vi "mirrorInterface.vi"(8 "error in (no error)":errorcluster, 11 "FPGA VI In":refnum<k20>) -> (0 "error out":errorcluster, 3 "FPGA VI Reference Out":refnum<k20>)   [LabVIEW 2016]
uses:
  controls/SocketServerStates.ctl
  <vilib>/Platform/TimedLoop/XDataNode/timing_clust.ctl
  <vilib>/Platform/TimedLoop/XDataNode/nitl_modes.ctl
  <vilib>/Platform/TimedLoop/XDataNode/wakeup.ctl
  <vilib>/Utility/error.llb/Error Cluster From Error Code.vi
  <vilib>/rvi/errors/niLvFpgaAdjustHostInterfaceError.vi
  <vilib>/platform/TimedLoop/XDataNode/XDataNode.xnode
  <vilib>/rvi/interface/nirviMethod/nirviMethod.xnode
  <vilib>/rvi/errors/niLvFpgaMergeErrorWithErrorCode.vi
  <vilib>/Platform/TimedLoop/XDataNode/XDNodeRunTimeDep.lvlib
  <vilib>/FPGAPlugInAG/Dynamic/niLvFpga_WriteFifo_Dynamic.vi
  controls/RT-Variables.lvlib
panel:
  out "bytes written 2":i32
  out "bytes written":i32
  out "length":i32
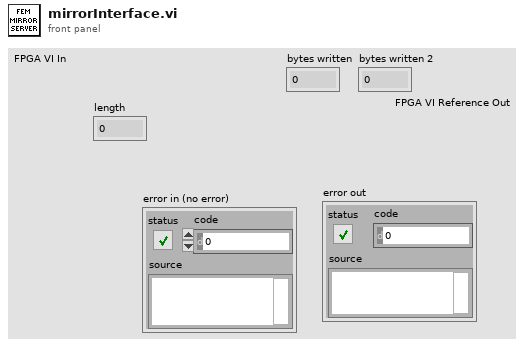
[diagram p1: front panel]
types:
  T1 = typedef "RT-Variables.lvlib/SocketServerStates.ctl" = enum16{"Wait", "SwitchState", "SingleUpdate", "ClosedLoop", "GetValues", "Exit"}
  T2 = typedef "XDNodeRunTimeDep.lvlib/timing_clust.ctl" = cluster{"Expected End [f-1]":u64, "Actual End [f-1]":u64, "Finished Late? [f-1]":bool, "Expected End [i-1]":u64, "Actual End [i-1]":u64, "Finished Late? [i-1]":bool, "Expected Start [i]":u64, "Actual Start [i]":u64, "Expected Start [f]":u64, "Actual Start [f]":u64, "Source Name":string, "Structure Name":string, "Period":i64, "Deadline":i64, "Offset":i64, "Start":i64, "Priority":i32, "Timeout":i32, "Mode":T3, "Wakeup Reason":T4, "Error":errorcluster, "Source Type":string, "Secondary Source Type":string, "Global End Time":u64, "Global Start Time":u64, "Frame Duration":u64, "Iteration Duration":u64, "Assigned CPU":i32, "I/O Scan Engine Mode":u32}
  T3 = typedef "XDNodeRunTimeDep.lvlib/nitl_modes.ctl" = enum32{"No Change", "Process missed periods, maintain original phase", "Discard missed periods, maintain original phase", "Process missed periods, ignore original phase", "Discard missed periods, ignore original phase"}
  T4 = typedef "XDNodeRunTimeDep.lvlib/wakeup.ctl" = enum32{"Normal", "Aborted", "Asynchronous wakeup", "Timing source error", "Timed loop error", "Timeout"}
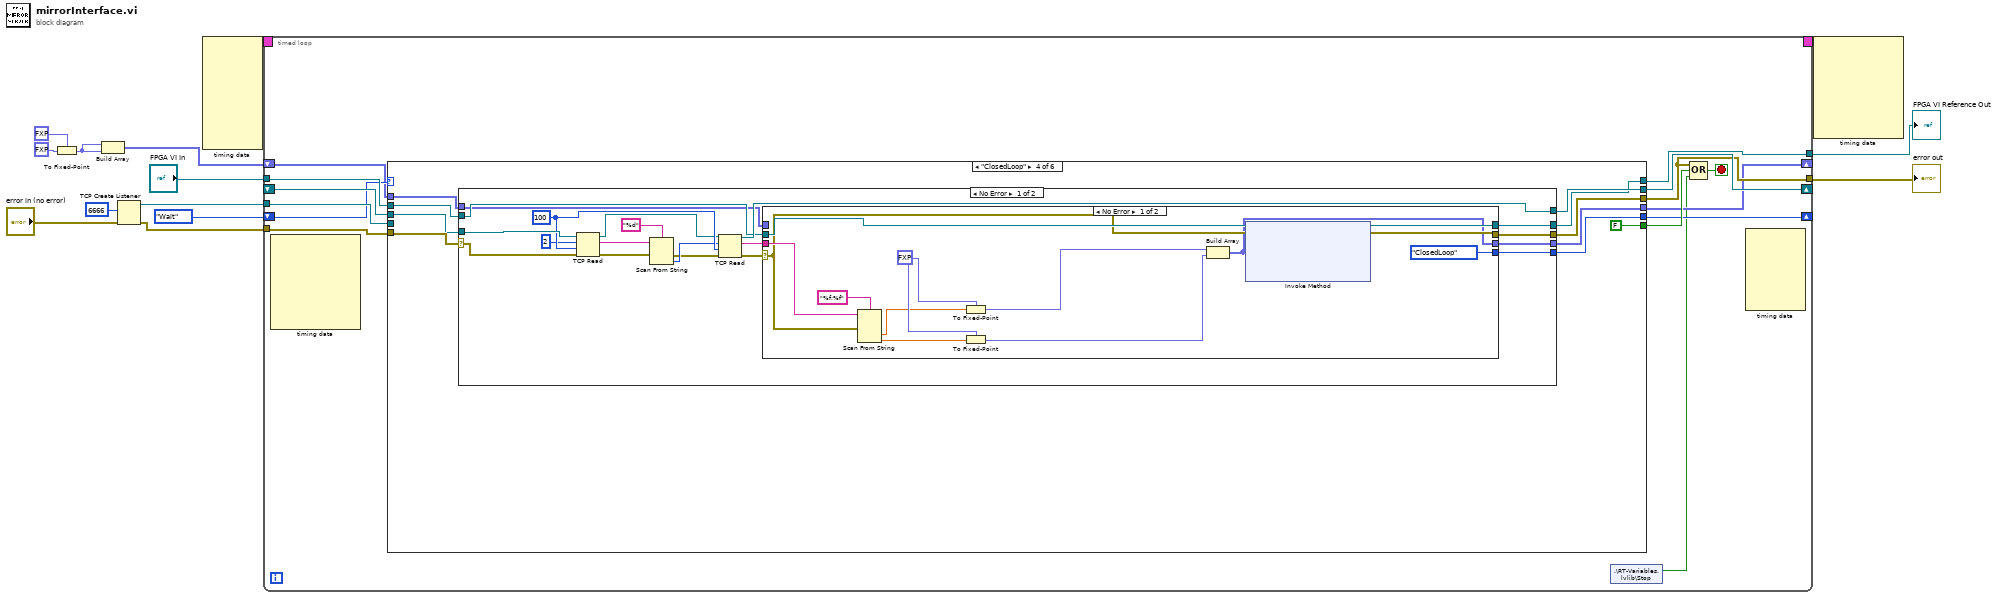
[diagram p0: block diagram]
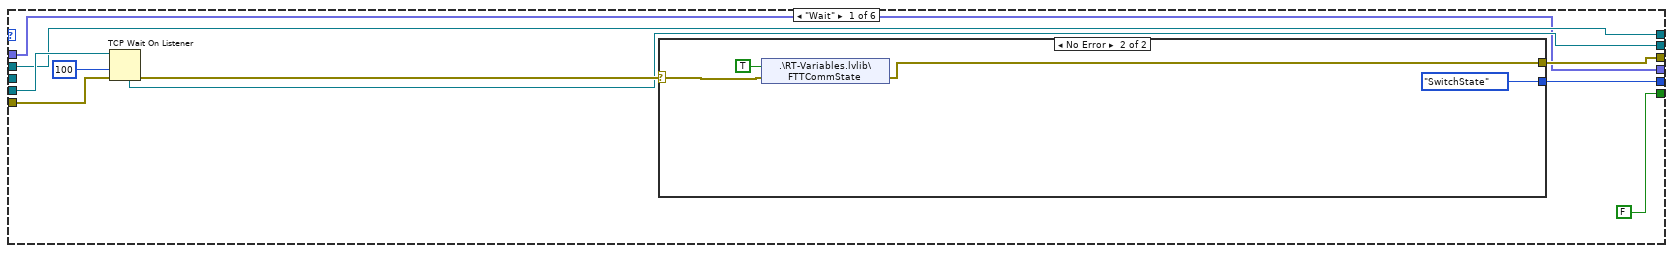
[diagram p2: hidden frame]
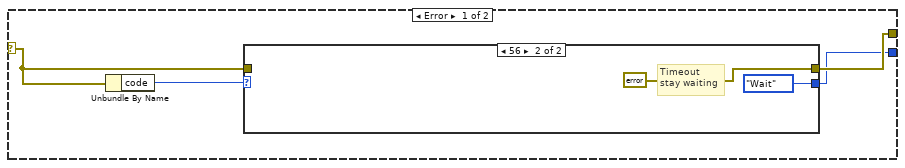
[diagram p3: hidden frame]
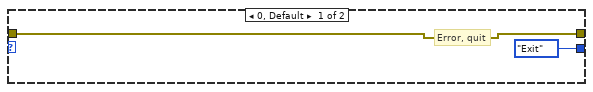
[diagram p4: hidden frame]
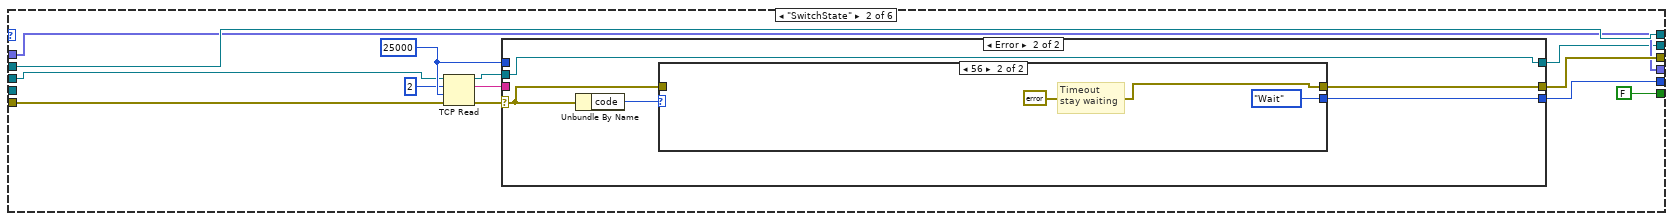
[diagram p5: hidden frame]
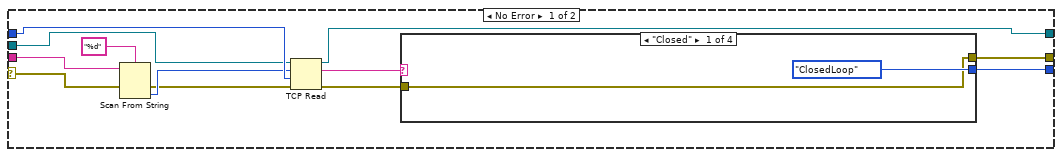
[diagram p6: hidden frame]
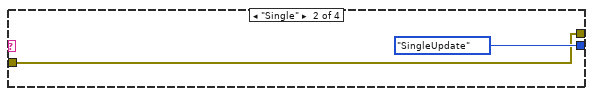
[diagram p7: hidden frame]
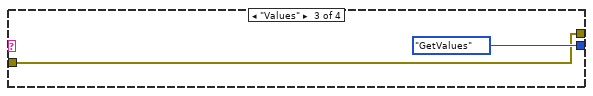
[diagram p8: hidden frame]
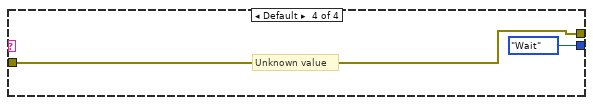
[diagram p9: hidden frame]
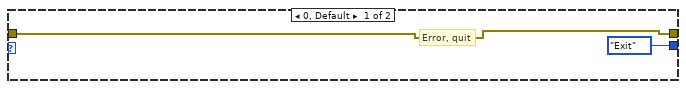
[diagram p10: hidden frame]
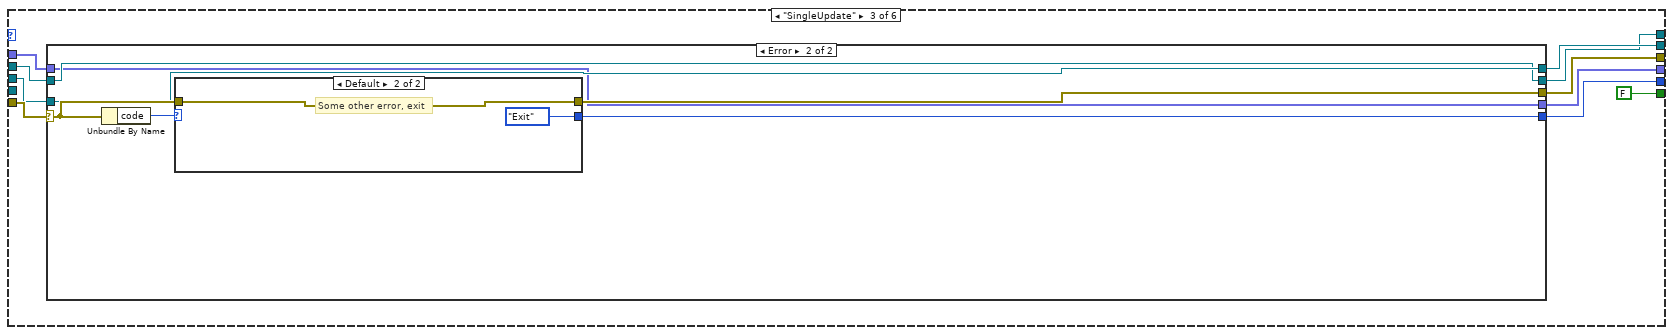
[diagram p11: hidden frame]
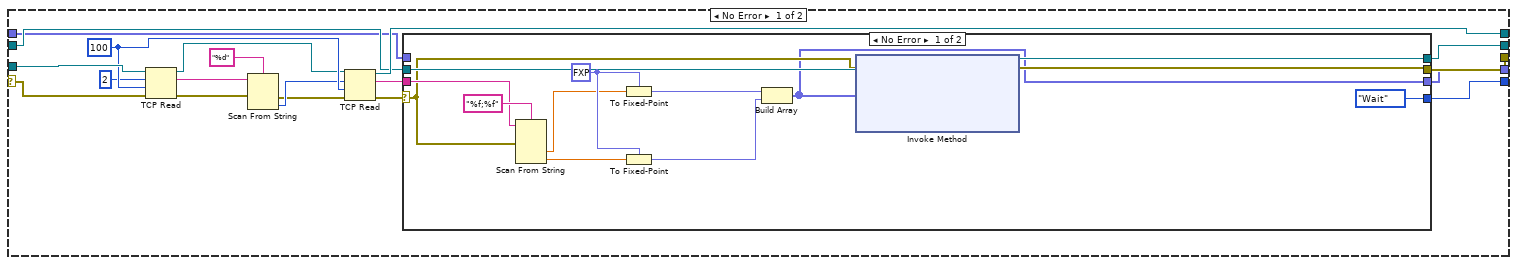
[diagram p12: hidden frame]
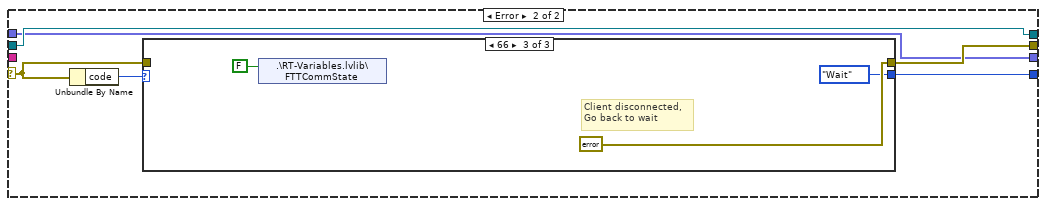
[diagram p13: hidden frame]
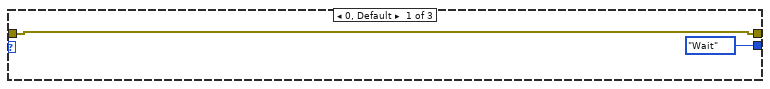
[diagram p14: hidden frame]
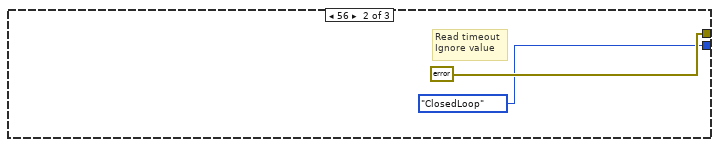
[diagram p15: hidden frame]
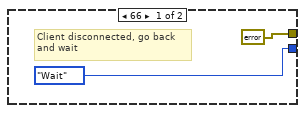
[diagram p16: hidden frame]
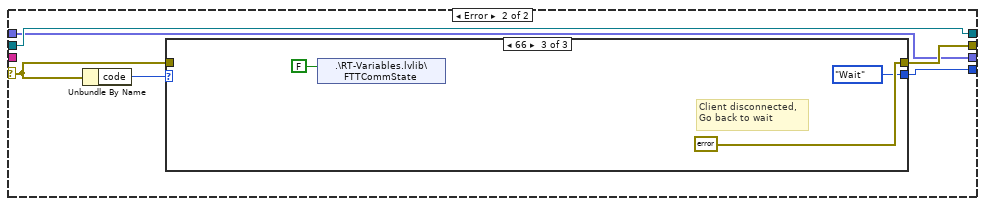
[diagram p17: hidden frame]
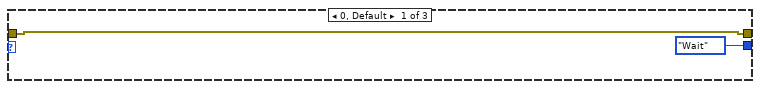
[diagram p18: hidden frame]
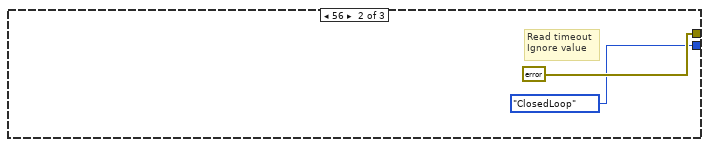
[diagram p19: hidden frame]
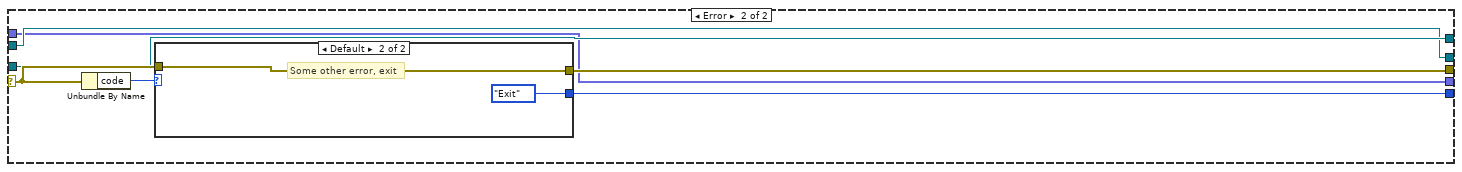
[diagram p20: hidden frame]
diagram:
  n1 = To Fixed-Point(fixed-point type=fxp<+/-,20,5> 0.0, number=fxp<+/-,32,16> 0.0) -> (fixed-point=w2:fxp<+/-,20,5>)
  n2 = Build Array(w2, w2) -> (w1:fxp<+/-,20,5>[])
  n3 = TCP Create Listener(8:"error in (no error)", 10:u16 6666 ("port")) -> (0:w8:errorcluster, 3:w13:refnum<k5>)  [unwired: 3 in, 1 out]
  n4 = node-c288() -> (w12:T2)  [unwired: 8 in]
  n5 = timed-loop {
    tunnel: w13 -> [w28]
    tunnel: w8 -> [w22]
    tunnel: "FPGA VI In" -> [w23]
    shift-right: [w27] -> _
    shift-left: _ -> [w26]
    timing: w12 -> [_]
    timing-out: [_] -> w11
    tunnel: [w21] -> w5
    tunnel: [w20] -> w10
    shift-right: [w19] -> _
    shift-left: SocketServerStates."Wait" -> [w18]
    shift-right: [w17] -> _
    shift-left: w1 -> [w16]
    stop <- w25 stop-if-true
    n6 = node-c288() -> ()  [unwired: 1 in, 7 out]
    n7 = case shown="\"ClosedLoop\"" w18 {
      tunnel: w22 -> [w37 w54 w102 w168 w226 w289]
      tunnel: w28 -> [w35 _ _ _ _ w290]
      tunnel: [w34 w61 w96 w167 w227 w288] -> w21
      tunnel: [w30 w63 w97 w166 w230 SocketServerStates."Exit"] -> w19
      tunnel: [w31 w52 w99 w164 w229 w291] -> w27
      tunnel: w26 -> [_ w53 w100 w165 w233 w291]
      tunnel: w23 -> [w32 w62 w101 w163 w232 w286]
      tunnel: [FALSE FALSE FALSE FALSE FALSE TRUE] -> w24
      tunnel: [w32 w62 w98 w161 w228 w286] -> w20
      tunnel: [w29 w60 w94 w159 w231 w284] -> w17
      tunnel: w16 -> [w29 w60 w93 w160 w234 w284]
      frame "Wait" {
        n8 = TCP Wait On Listener(8:w37, 9:100 ("timeout ms (wait forever: -1)"), 11:w35) -> (0:w36:errorcluster, 4:w31:refnum<k5>)  [unwired: 1 in, 3 out]
        n9 = case shown="No Error" w36 {
          selector: w36 -> [w40 w48]
          tunnel: [w41 w49] -> w34
          tunnel: [w39 SocketServerStates."SwitchState"] -> w30
          frame Error {
            n10 = Unbundle By Name(w40) -> ("code"=w42:i32)
            n11 = case shown="56" w42 {
              tunnel: [w44 errorcluster {"status"=FALSE, "code"=0, "source"=""} ("error constant")] -> w41
              tunnel: w40 -> [w44 _]
              tunnel: [SocketServerStates."Exit" SocketServerStates."Wait"] -> w39
              frame 0, Default {
                # "Error, quit"
              }
              frame 56 {
                # "Timeout\nstay waiting"
              }
            }
          }
          frame No Error {
            n12 = shared-variable ".\\RT-Variables.lvlib\\FTTCommState"(TRUE ("FTTCommState"), error in=w48) -> (error out=w49:errorcluster)
          }
        }
      }
      frame "SwitchState" {
        w58 = 25000 ("timeout ms (25000)")
        n13 = TCP Read(connection ID=w53, bytes to read=2, error in (no error)=w54, 9:w58) -> (connection ID out=w56:refnum<k5>, data out=w57:string, error out=w51:errorcluster)  [unwired: 1 in]
        n14 = case shown="Error" w51 {
          selector: w51 -> [w64 w87]
          tunnel: [w75 w86] -> w63
          tunnel: [w74 w85] -> w61
          tunnel: w58 -> [w73 _]
          tunnel: w57 -> [w70 _]
          tunnel: w56 -> [w69 w84]
          tunnel: [w65 w84] -> w52
          frame No Error {
            n15 = Scan From String(format string="%d", input string=w70, error in=w64) -> (error out=w71:errorcluster, output 1=w72:i32)  [unwired: 2 in, 2 out]
            n16 = TCP Read(connection ID=w69, bytes to read=w72, error in (no error)=w71, 9:w73) -> (connection ID out=w65:refnum<k5>, data out=w66:string, error out=w67:errorcluster)  [unwired: 1 in]
            n17 = case shown="\"Closed\"" w66 {
              tunnel: [SocketServerStates."ClosedLoop" SocketServerStates."SingleUpdate" SocketServerStates."GetValues" SocketServerStates."Wait"] -> w75
              tunnel: w67 -> [w76 w78 w80 w83]
              tunnel: [w76 w78 w80 w83] -> w74
              frame "Closed" {
              }
              frame "Single" {
              }
              frame "Values" {
              }
              frame Default {
                # "Unknown value"
              }
            }
          }
          frame Error {
            n18 = Unbundle By Name(w87) -> ("code"=w88:i32)
            n19 = case shown="56" w88 {
              tunnel: [w90 errorcluster {"status"=FALSE, "code"=0, "source"=""} ("error constant")] -> w85
              tunnel: w87 -> [w90 _]
              tunnel: [SocketServerStates."Exit" SocketServerStates."Wait"] -> w86
              frame 0, Default {
                # "Error, quit"
              }
              frame 56 {
                # "Timeout\nstay waiting"
              }
            }
          }
        }
      }
      frame "SingleUpdate" {
        n20 = case shown="Error" w102 {
          selector: w102 -> [w114 w153]
          tunnel: [w120 w152] -> w96
          tunnel: [w116 w151] -> w97
          tunnel: w100 -> [w113 w150]
          tunnel: [w118 w150] -> w99
          tunnel: w101 -> [w117 w149]
          tunnel: [w115 w149] -> w98
          tunnel: [w104 w148] -> w94
          tunnel: w93 -> [w103 w148]
          frame No Error {
            w112 = 100 ("timeout ms (25000)")
            n21 = TCP Read(connection ID=w113, bytes to read=2, error in (no error)=w114, 9:w112) -> (connection ID out=w107:refnum<k5>, data out=w108:string, error out=w111:errorcluster)  [unwired: 1 in]
            n22 = Scan From String(format string="%d", input string=w108, error in=w111) -> (error out=w109:errorcluster, output 1=w110:i32)  [unwired: 2 in, 2 out]
            n23 = TCP Read(connection ID=w107, bytes to read=w110, error in (no error)=w109, 9:w112) -> (connection ID out=w118:refnum<k5>, data out=w119:string, error out=w121:errorcluster)  [unwired: 1 in]
            n24 = case shown="No Error" w121 {
              selector: w121 -> [w127 w139]
              tunnel: [w126 w138] -> w120
              tunnel: w119 -> [w133 _]
              tunnel: w117 -> [w129 w136]
              tunnel: [SocketServerStates."Wait" w137] -> w116
              tunnel: [w128 w136] -> w115
              tunnel: [w122 w135] -> w104
              tunnel: w103 -> [_ w135]
              frame No Error {
                w132 = fxp<+/-,20,5> 0.0 ("fixed-point type")
                n25 = Scan From String(format string="%f;%f", input string=w133, error in=w127) -> (output 1=w125:dbl, output 2=w124:dbl)  [unwired: 3 in, 3 out]
                n26 = To Fixed-Point(fixed-point type=w132, number=w125) -> (fixed-point=w131:fxp<+/-,20,5>)
                n27 = To Fixed-Point(fixed-point type=w132, number=w124) -> (fixed-point=w130:fxp<+/-,20,5>)
                n28 = Build Array(w131, w130) -> (w122:fxp<+/-,20,5>[])
                n29 = xnode "Invoke Method"("FPGA VI Reference In"=w129, "error in"=w127, "Data"=w122) -> ("FPGA VI Reference Out"=w128:refnum<k20>, "error out"=w126:errorcluster)  [unwired: 1 in, 1 out]
              }
              frame Error {
                n30 = Unbundle By Name(w139) -> ("code"=w140:i32)
                n31 = case shown="66" w140 {
                  tunnel: w139 -> [w142 _ _]
                  tunnel: [w142 errorcluster {"status"=FALSE, "code"=0, "source"=""} ("error constant") errorcluster {"status"=FALSE, "code"=0, "source"=""} ("error constant")] -> w138
                  tunnel: [SocketServerStates."Wait" SocketServerStates."ClosedLoop" SocketServerStates."Wait"] -> w137
                  frame 0, Default {
                  }
                  frame 56 {
                    # "Read timeout\nIgnore value"
                  }
                  frame 66 {
                    # "Client disconnected,\nGo back to wait"
                    n32 = shared-variable ".\\RT-Variables.lvlib\\FTTCommState"(FALSE ("Cal. Mirror")) -> ()  [unwired: 1 in, 1 out]
                  }
                }
              }
            }
          }
          frame Error {
            n33 = Unbundle By Name(w153) -> ("code"=w154:i32)
            n34 = case shown="Default" w154 {
              tunnel: w153 -> [_ w158]
              tunnel: [errorcluster {"status"=FALSE, "code"=0, "source"=""} ("error constant") w158] -> w152
              tunnel: [SocketServerStates."Wait" SocketServerStates."Exit"] -> w151
              frame 66 {
                # "Client disconnected, go back\nand wait"
              }
              frame Default {
                # "Some other error, exit"
              }
            }
          }
        }
      }
      frame "ClosedLoop" {
        n35 = case shown="No Error" w168 {
          selector: w168 -> [w180 w219]
          tunnel: [w186 w218] -> w167
          tunnel: [w182 w217] -> w166
          tunnel: w165 -> [w179 w216]
          tunnel: [w184 w216] -> w164
          tunnel: w163 -> [w183 w215]
          tunnel: [w181 w215] -> w161
          tunnel: w160 -> [w170 w214]
          tunnel: [w169 w214] -> w159
          frame No Error {
            w178 = 100 ("timeout ms (25000)")
            n36 = TCP Read(connection ID=w179, bytes to read=2, error in (no error)=w180, 9:w178) -> (connection ID out=w173:refnum<k5>, data out=w174:string, error out=w177:errorcluster)  [unwired: 1 in]
            n37 = Scan From String(format string="%d", input string=w174, error in=w177) -> (error out=w175:errorcluster, output 1=w176:i32)  [unwired: 2 in, 2 out]
            n38 = TCP Read(connection ID=w173, bytes to read=w176, error in (no error)=w175, 9:w178) -> (connection ID out=w184:refnum<k5>, data out=w185:string, error out=w187:errorcluster)  [unwired: 1 in]
            n39 = case shown="No Error" w187 {
              selector: w187 -> [w195 w205]
              tunnel: [w194 w204] -> w186
              tunnel: w185 -> [w199 _]
              tunnel: w183 -> [w197 w202]
              tunnel: [SocketServerStates."ClosedLoop" w203] -> w182
              tunnel: [w196 w202] -> w181
              tunnel: w170 -> [_ w201]
              tunnel: [w192 w201] -> w169
              frame No Error {
                w198 = fxp<+/-,20,5> 0.0 ("fixed-point type")
                n40 = Scan From String(format string="%f;%f", input string=w199, error in=w195) -> (output 1=w190:dbl, output 2=w191:dbl)  [unwired: 3 in, 3 out]
                n41 = To Fixed-Point(fixed-point type=w198, number=w190) -> (fixed-point=w189:fxp<+/-,20,5>)
                n42 = To Fixed-Point(fixed-point type=w198, number=w191) -> (fixed-point=w188:fxp<+/-,20,5>)
                n43 = Build Array(w189, w188) -> (w192:fxp<+/-,20,5>[])
                n44 = xnode "Invoke Method"("FPGA VI Reference In"=w197, "error in"=w195, "Data"=w192) -> ("FPGA VI Reference Out"=w196:refnum<k20>, "error out"=w194:errorcluster)  [unwired: 1 in, 1 out]
              }
              frame Error {
                n45 = Unbundle By Name(w205) -> ("code"=w206:i32)
                n46 = case shown="66" w206 {
                  tunnel: w205 -> [w208 _ _]
                  tunnel: [w208 errorcluster {"status"=FALSE, "code"=0, "source"=""} ("error constant") errorcluster {"status"=FALSE, "code"=0, "source"=""} ("error constant")] -> w204
                  tunnel: [SocketServerStates."Wait" SocketServerStates."ClosedLoop" SocketServerStates."Wait"] -> w203
                  frame 0, Default {
                  }
                  frame 56 {
                    # "Read timeout\nIgnore value"
                  }
                  frame 66 {
                    # "Client disconnected,\nGo back to wait"
                    n47 = shared-variable ".\\RT-Variables.lvlib\\FTTCommState"(FALSE ("Cal. Mirror")) -> ()  [unwired: 1 in, 1 out]
                  }
                }
              }
            }
          }
          frame Error {
            n48 = Unbundle By Name(w219) -> ("code"=w220:i32)
            n49 = case shown="Default" w220 {
              tunnel: w219 -> [_ w224]
              tunnel: [errorcluster {"status"=FALSE, "code"=0, "source"=""} ("error constant") w224] -> w218
              tunnel: [SocketServerStates."Wait" SocketServerStates."Exit"] -> w217
              frame 66 {
                # "Client disconnected, go back\nand wait"
              }
              frame Default {
                # "Some other error, exit"
              }
            }
          }
        }
      }
      frame "GetValues" {
        n50 = case shown="No Error" w226 {
          selector: w226 -> [w241 w278]
          tunnel: [w242 w277] -> w227
          tunnel: [w243 w276] -> w230
          tunnel: w233 -> [w255 w275]
          tunnel: [w251 w275] -> w229
          tunnel: w232 -> [w240 w274]
          tunnel: [w240 w274] -> w228
          tunnel: [w239 w273] -> w231
          tunnel: w234 -> [w239 w273]
          frame No Error {
            w258 = "" ("initial string")
            w250 = 25000 ("timeout ms (25000)")
            n51 = Index Array(array=w239, index #1=0 ("index"), index #2=1 ("index")) -> (element #1=w236:fxp<+/-,20,5>, element #2=w235:fxp<+/-,20,5>)
            n52 = To Single Precision Float(number=w236) -> (single precision float=w261:sgl)
            n53 = To Single Precision Float(number=w235) -> (single precision float=w260:sgl)
            n54 = Format Into String(format string="%f;%f", initial string=w258, error in=w241, w261, w260) -> (resulting string=w249:string, error out=w257:errorcluster)
            n55 = String Length(string=w249) -> (length=w259:i32)
            n56 = Format Into String(format string="%2d", initial string=w258, error in=w257, w259) -> (resulting string=w248:string, error out=w254:errorcluster)
            n57 = String Length(string=w248) -> (length=→"length":i32)
            n58 = TCP Write(connection ID=w255, data in=w248, error in (no error)=w254, 9:w250) -> (connection ID out=w252:refnum<k5>, bytes written=→"bytes written":i32, error out=w253:errorcluster)
            n59 = TCP Write(connection ID=w252, data in=w249, error in (no error)=w253, 9:w250) -> (connection ID out=w251:refnum<k5>, bytes written=→"bytes written 2":i32, error out=w244:errorcluster)
            n60 = case shown="No Error" w244 {
              selector: w244 -> [w263 w267]
              tunnel: [SocketServerStates."Wait" w268] -> w243
              tunnel: [w263 w265] -> w242
              frame No Error {
              }
              frame Error {
                n61 = Unbundle By Name(w267) -> ("code"=w266:i32)
                n62 = case shown="66" w266 {
                  tunnel: [SocketServerStates."Exit" SocketServerStates."Wait"] -> w268
                  tunnel: [errorcluster {"status"=FALSE, "code"=0, "source"=""} ("error constant") errorcluster {"status"=FALSE, "code"=0, "source"=""} ("error constant")] -> w265
                  frame 0, Default {
                  }
                  frame 66 {
                    # "Timeout"
                  }
                }
              }
            }
          }
          frame Error {
            n63 = Unbundle By Name(w278) -> ("code"=w279:i32)
            n64 = case shown="66" w279 {
              tunnel: w278 -> [_ _]
              tunnel: [errorcluster {"status"=FALSE, "code"=0, "source"=""} ("error constant") errorcluster {"status"=FALSE, "code"=0, "source"=""} ("error constant")] -> w277
              tunnel: [SocketServerStates."Wait" SocketServerStates."Exit"] -> w276
              frame 66 {
                # "Client disconnected, go back\nand wait"
              }
              frame Default {
                # "Some other error, exit"
              }
            }
          }
        }
      }
      frame "Exit", Default {
        n65 = TCP Close Connection(connection ID=w290, error in (no error)=w289) -> (error out=w288:errorcluster)  [unwired: 1 in, 1 out]
      }
    }
    n66 = shared-variable ".\\RT-Variables.lvlib\\Stop"() -> (w15:bool)  [unwired: 1 in, 1 out]
    n67 = Compound Arithmetic op=OR(w21, w24, w15) -> (w25:bool)
    n68 = node-c288() -> ()  [unwired: 6 in, 1 out]
  }
  "error out" <- w5
  "FPGA VI Reference Out" <- w10
  n69 = node-c288(w11) -> ()  [unwired: 7 out]
